vi "testWrongDataSet.vi"() -> ()   [LabVIEW 2019, in "TestCaseTest.lvlib" / "Theory.lvlib"]
uses:
  Theory.lvlib
  TestCaseTestSupport/FakeTheory.vi
  TestCase/Theory/Theory.lvclass
  TestCaseTestSupport/TestCaseTestSupport.lvlib
  Assertion/Assertion.lvlib
panel:
  out "error out":errorcluster
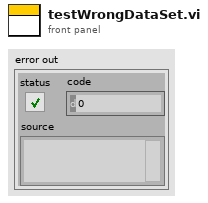
[diagram p1: front panel]
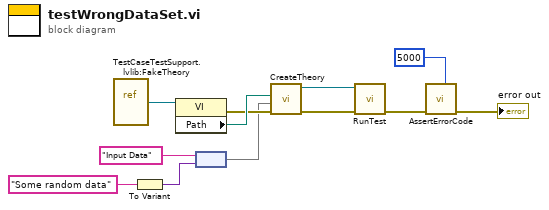
[diagram p0: block diagram]
diagram:
  n1 = vi-ref "TestCaseTestSupport.lvlib:FakeTheory.vi"() -> (w10:refnum<vi>)
  n2 = To Variant(anything="Some random data" ("key")) -> (Variant=w2:variant)
  n3 = property class="VI"(reference=w10) -> (error out=w8:errorcluster, "Path"=w9:path)  [unwired: 1 in, 1 out]
  n4 = node("Input Data" ("key"), w2) -> (w3:map{string, variant})
  n5 = call "CreateTheory.vi"("error in (no error)"=w8, "Control Data"=w3, "Path"=w9) -> ("error out"=w11:errorcluster, "Theory"=w12:refnum<class "Theory.lvclass">)  [unwired: 7 in]
  n6 = call-dynamic "RunTest.vi"("error in (no error)"=w11, "Theory in"=w12) -> ("error out"=w7:errorcluster)  [unwired: 8 in, 1 out]
  n7 = call "AssertErrorCode.vi"("Expected"=5000, "error in (no error)"=w7) -> ("error out"=→"error out":errorcluster)  [unwired: 9 in]
